vi "Triaxial_Geonor_General.vi"() -> ()   [LabVIEW 2015]
uses:
  <vilib>/Analysis/Matrix/Datatypes/RealMatrix.ctl
  <vilib>/Utility/file.llb/Read From Spreadsheet File (DBL).vi
  <vilib>/Analysis/Matrix/Numeric/Conversions/Array To Matrix - RA.vi
  Variables_Offset.vi
  <vilib>/Analysis/Matrix/NI_Matrix.lvlib
panel:
  in  "BoolSat":bool=TRUE
  in  "BoolBCh":bool=TRUE
  in  "BoolCons":bool=TRUE
  in  "BoolCD":bool=TRUE
  in  "BoolUU":bool=TRUE
  in  "BoolCU":bool=TRUE
  out "Vect Prom Efec":bool
  out "OUTPUT":i32[](array[numeric])
  out "w_4":dbl[][](array[numeric])
  out "w_3s":dbl[][](array[numeric])
  out "Vec_Esfuerzo_principal":dbl[](array[numeric]) format="%.2f"
  out "Vec_Desviador":dbl[](array[numeric]) format="%.2f"
  out "Vec_Promedio_efectivo":dbl[](array[numeric]) format="%.2f"
  out "Vec_Esfuerzo_prom_princ":dbl[](array[numeric]) format="%.2f"
  out "Vec_Esfuerzo_radial":dbl[](array[numeric]) format="%.2f"
  out "Vec_AreaCorr":dbl[](array[numeric]) format="%.2f"
  out "Vec_Deformacionporc":dbl[](array[numeric]) format="%.2f"
  in  "Falla CD":bool
  in  "Falla UU":bool
  in  "Falla CU":bool
  in  "B-Check":bool
  out "Log_tiempo [seg]":ext
  out "Raiz_tiempo [seg]":ext
  out "Tiempo Total[s]":ext
  in  "INICIO":bool
  out "vector B Skepton":dbl[](array[numeric]) format="%.2f"
  out "offset 11":dbl
  out "PresionVol":dbl
  out "LVDT Volumen":bool
  out "LVDT Axial":bool
  out "P. Poros":bool
  out "P. Camara":bool
  out "Celda Carga":bool
  out "vector desp vol":dbl[](array[numeric]) format="%.2f"
  out "TIME RAIZ":dbl[](array[numeric]) format="%.2f"
  out "TIME LOG":dbl[](array[numeric]) format="%.2f"
  out "offset 10":dbl
  out "PresCamara":dbl
  out "offset 9":dbl
  out "PresPoro":dbl
  in  "Consolidación":bool
  in  "Saturación":bool
  out "Boolean":bool
  out "offset 8":dbl
  out "offset 7":dbl
  in  "Offset":bool
  out "Cvol":dbl
  out "Ccarga":dbl
  out "Clvdtax":dbl
  out "Ccamara":dbl
  out "Cporo":dbl
  out "Pvol":dbl
  out "Pcarga":dbl
  out "Plvdtax":dbl
  out "Pcamara":dbl
  out "Pporo":dbl
  out "all rows":dbl[][](array[numeric])
  out "vector poros":dbl[](array[numeric]) format="%.2f"
  out "vector camara":dbl[](array[numeric]) format="%.2f"
  out "vector carga":dbl[](array[numeric]) format="%.2f"
  out "vector desp axial":dbl[](array[numeric]) format="%.2f"
  out "LVDT_AX":dbl
  out "Carga":dbl
  in  "Tab Control":T1(tab)
  in  "Peso [g]":string
  out "Fallando":bool
  out "Consolidando":bool
  out "Saturando":bool
  in  "Muestreo Falla":dbl
  in  "Muestreo Consolidación":dbl
  in  "Muestreo Saturación":dbl
  out "Tiempo Falla [s]":dbl
  out "Tiempo Consolidación [s]":dbl
  out "Tiempo Saturación [s]":dbl
  out "Etapa Actual":string
  in  "Diametro [mm]":string
  in  "Altura [mm]":string
  in  "Filename":path=path "Consolidacion"
  out "path":path
  out "Index":dbl
  out "Cambio de Volumen [mm^3]":dbl(slide) scale=0.0..60.0 scale format="%#_3f"
  out "Presión de Poros [KPa]":dbl(knob) scale=0.0..450.0 scale format="%#_3p"
  out "Desplazamiento Axial [mm]":dbl(slide) scale=0.0..15.0 scale format="%.0p"
  out "Celda de Carga [N]":dbl(knob) scale=0.0..300.0 scale format="%_2p"
  out "Presión de Camara [KPa]":dbl(knob) scale=0.0..450.0 scale format="%#_1f"
  out "B Skempton":dbl
  out "Parametro B camara":dbl
  out "Parametro B Poros":dbl
  in  "Fijar Presiones":bool
  in  "Tab Control 2":enum32{"Grafica A", "Grafica B", "Grafica C"}(tab)
  out "Grafica A":cluster{"X":dbl[], "Y":dbl[]}[](graph)
  in  "OK Button":bool
  out "Grafica B":cluster{"X":dbl[], "Y":dbl[]}[](graph)
  in  "OK Button 2":bool
  out "Grafica C":cluster{"X":dbl[], "Y":dbl[]}[](graph)
  in  "OK Button 3":bool
  in  "Grafica A - Valores en X":string(combo)
  in  "Grafica A - Valores en Y":string(combo)
  in  "Grafica B - Valores en X":string(combo)
  in  "Grafica B - Valores en Y":string(combo)
  in  "Grafica C - Valores en X":string(combo)
  in  "Grafica C - Valores en Y":string(combo)
  out "Error":dbl
  in  "Velocidad mm/min":dbl
  out "V_max":dbl
  out "V_min":dbl
  out "Velocidades":dbl[][](array[numeric])
  out "INPUT":i32[](array[numeric])
  out "OUTPUT":T2
  out "TIME SEC":dbl[](array[numeric]) format="%.2f"
  out "Boolean 2":bool
  out "Tiempo [min]":dbl format="%#_1g"
  in  "stop":bool
  in  "Conect":bool
  # "MOD SAT-CON"
  # "MOD FALLAS"
  # "Sensores Activos"
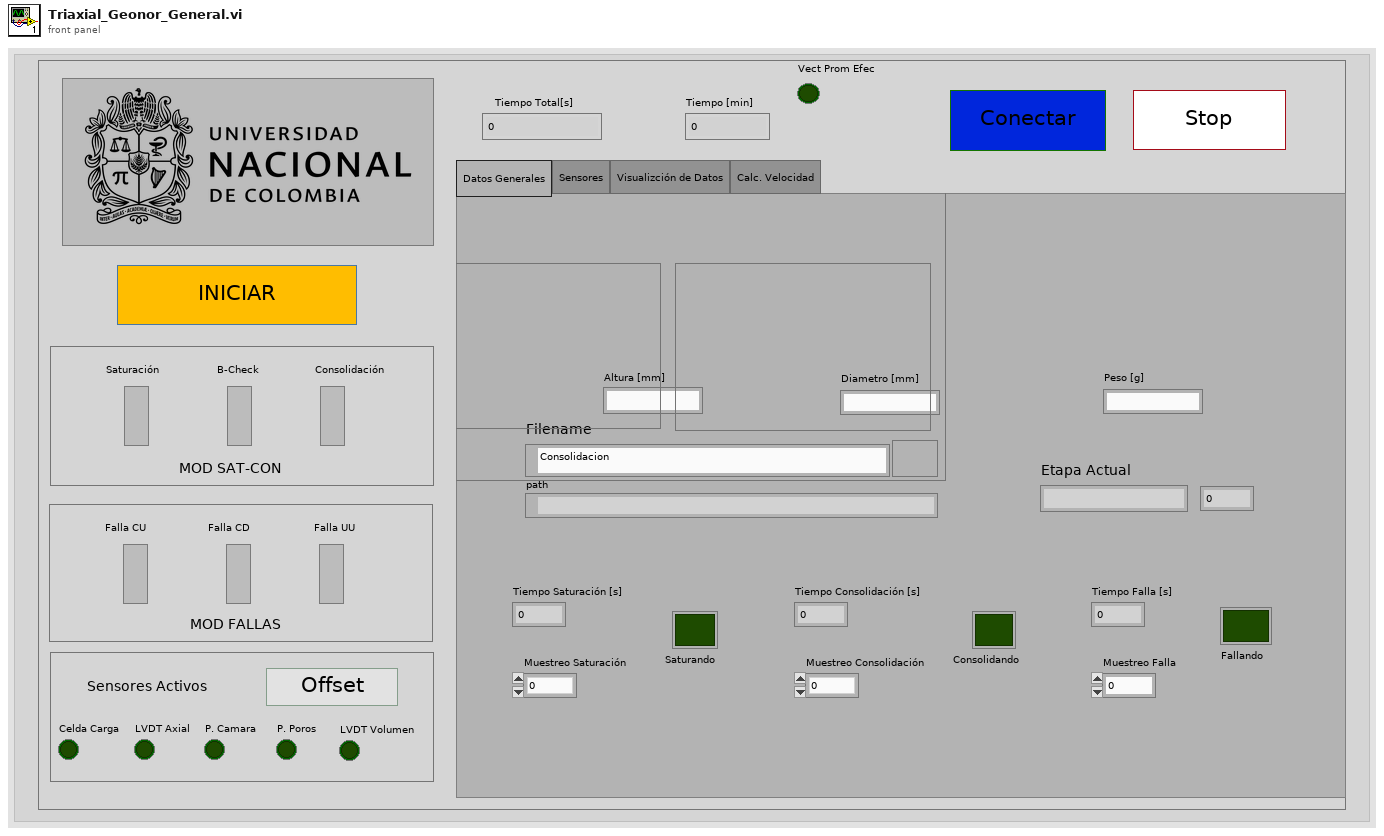
[diagram p1: front panel]
types:
  T1 = enum32{"Datos Generales", "Sensores", "Visualizción de Datos", "Calc. Velocidad"}
  T2 = typedef "NI_Matrix.lvlib/RealMatrix.ctl" = dbl[][]
  T3 = enum16{"open", "open or create", "create or replace", "create", "open (read-only)"}
diagram:
  n1 = flat-sequence {
    frame #0 {
      n2 = while {
        stop <- "Conect" stop-if-true
        n3 = local read "Boolean"() -> (→"Boolean":bool)
      }
      n4 = call "Display Message to User"() -> ()  [unwired: 10 in, 2 out]
      n5 = property on="Tab Control" class="TabCtl (strict)"("PaneHeight"=605) -> (error out=w1:errorcluster)  [unwired: 2 in, 1 out]
      n6 = property on="Tab Control" class="TabCtl (strict)"(error in=w1, "PaneWidth"=890) -> ()  [unwired: 1 in, 2 out]
    }
    frame #1 {
      w8 = FALSE
      w6 = 0.0
      n7 = Initialize Array(0.0, 0 ("dimension size")) -> (→"TIME SEC" →"vector desp axial" →"vector carga" →"vector camara" →"vector poros" →"TIME LOG" →"TIME RAIZ" →"vector desp vol" →"vector B Skepton" →"Vec_Deformacionporc" →"Vec_AreaCorr" →"Vec_Esfuerzo_radial" →"Vec_Esfuerzo_prom_princ" →"Vec_Promedio_efectivo" →"Vec_Desviador" →"Vec_Esfuerzo_principal":dbl[])
      n8 = local write "Saturación"(w8) -> ()
      n9 = local write "Consolidación"(w8) -> ()
      n10 = local write "Falla CU"(w8) -> ()
      n11 = local write "LVDT Axial"(w8) -> ()
      n12 = local write "LVDT Volumen"(w8) -> ()
      n13 = local write "B-Check"(w8) -> ()
      n14 = local write "Celda Carga"(w8) -> ()
      n15 = local write "Consolidando"(w8) -> ()
      n16 = local write "Saturando"(w8) -> ()
      n17 = local write "Falla UU"(w8) -> ()
      n18 = local write "Falla CD"(w8) -> ()
      n19 = local write "Boolean 2"(w8) -> ()
      n20 = local write "P. Camara"(w8) -> ()
      n21 = local write "P. Poros"(w8) -> ()
      n22 = local write "Fallando"(w8) -> ()
      n23 = local write "Parametro B Poros"(w6) -> ()
      n24 = local write "Parametro B camara"(w6) -> ()
      n25 = local write "offset 11"(w6) -> ()
      n26 = local write "offset 7"(w6) -> ()
      n27 = local write "offset 9"(w6) -> ()
      n28 = local write "offset 10"(w6) -> ()
      n29 = local write "B Skempton"(w6) -> ()
      n30 = local write "offset 8"(w6) -> ()
      "Index" <- w6
    }
    frame #2 {
      w16 = ext 0.0 ("x-y*floor(x/y)")
      n31 = Wait (ms)(milliseconds to wait=u32 1000) -> ()  [unwired: 1 out]
      n32 = local write "Tiempo Total[s]"(w16) -> ()
      n33 = local write "Tiempo Consolidación [s]"(w16) -> ()
      n34 = local write "Tiempo Falla [s]"(w16) -> ()
      n35 = local write "Tiempo Saturación [s]"(w16) -> ()
      n36 = Path To String(path="Filename") -> (string=w62:string)
      n37 = Concatenate Strings("C:\\Users\\LAB GEOTECNIA UN IEI\\Desktop\\GEONOR\\GEONOR\\Datos_Ensayo\\", w62) -> (w61:string)
      n38 = String To Path(string=w61) -> (path=w59:path)
      "path" <- w59
      n39 = call-poly <vilib>:"Read From Spreadsheet File.vi"("file path (dialog if empty)"=path "C:/Users/LAB GEOTECNIA UN IEI/Desktop/GEONOR/GEONOR/Archivo_de_calibración.txt") -> ("all rows"=w18:dbl[][])  [unwired: 6 in, 4 out]
      "all rows" <- w18
      n40 = TDMS Open(10:T3."create" ("operation (0:open)"), 11:w59) -> (0:w55:errorcluster, 3:w56:refnum<k34>)  [unwired: 5 in]
      n41 = flat-sequence {
        tunnel: [w69] -> w22
        tunnel: [w68] -> w21
        tunnel: w56 -> [w67]
        tunnel: w55 -> [w66]
        tunnel: w22 -> [w75]
        tunnel: [w74] -> w20
        tunnel: w21 -> [w72]
        tunnel: [w73] -> w19
        tunnel: w20 -> [w81]
        tunnel: [w80] -> w15
        tunnel: w19 -> [w79]
        tunnel: [w78] -> w14
        tunnel: w15 -> [w85]
        tunnel: w14 -> [w87]
        tunnel: [w86] -> w13
        tunnel: [w84] -> w12
        tunnel: w13 -> [w89]
        tunnel: w12 -> [w88]
        frame #0 {
          n42 = TDMS Set Properties(5:"Laboratorio de Geotecnia" ("property name"), 7:"Author" ("property name"), 8:w66, 11:w67) -> (0:w68:errorcluster, 3:w69:refnum<k34>)  [unwired: 2 in, 2 out]
        }
        frame #1 {
          n43 = TDMS Set Properties(5:"Altura [mm]", 7:"Altura [mm]", 8:w72, 11:w75) -> (0:w73:errorcluster, 3:w74:refnum<k34>)  [unwired: 2 in, 2 out]
        }
        frame #2 {
          n44 = TDMS Set Properties(5:"Diametro [mm]", 7:"Diametro [mm]", 8:w79, 11:w81) -> (0:w78:errorcluster, 3:w80:refnum<k34>)  [unwired: 2 in, 2 out]
        }
        frame #3 {
          n45 = TDMS Set Properties(5:"Peso [g]", 7:"Peso [gr]", 8:w87, 11:w85) -> (0:w86:errorcluster, 3:w84:refnum<k34>)  [unwired: 2 in, 2 out]
        }
        frame #4 {
          n46 = TDMS Close(8:w89, 11:w88) -> ()  [unwired: 2 out]
        }
      }
      n47 = Index Array(array=w18, index (row)=1, index (col)=2 ("disabled index (col)")) -> (element=→"Cporo":dbl)
      n48 = Index Array(array=w18, index (row)=1, index (col)=1 ("disabled index (col)")) -> (element=→"Pporo":dbl)
      n49 = Index Array(array=w18, index (row)=2, index (col)=2 ("disabled index (col)")) -> (element=→"Ccamara":dbl)
      n50 = Index Array(array=w18, index (row)=2, index (col)=1 ("disabled index (col)")) -> (element=→"Pcamara":dbl)
      n51 = Index Array(array=w18, index (row)=3, index (col)=2 ("disabled index (col)")) -> (element=→"Clvdtax":dbl)
      n52 = Index Array(array=w18, index (row)=3, index (col)=1 ("disabled index (col)")) -> (element=→"Plvdtax":dbl)
      n53 = Index Array(array=w18, index (row)=4, index (col)=1 ("disabled index (col)")) -> (element=→"Pcarga":dbl)
      n54 = Index Array(array=w18, index (row)=5, index (col)=2 ("disabled index (col)")) -> (element=→"Cvol":dbl)
      n55 = Index Array(array=w18, index (row)=5, index (col)=1 ("disabled index (col)")) -> (element=→"Pvol":dbl)
      n56 = Index Array(array=w18, index (row)=4, index (col)=2 ("disabled index (col)")) -> (element=→"Ccarga":dbl)
      "Boolean 2" <- TRUE
      "Etapa Actual" <- "Esperando Inicio"
      "Error" <- 0.005
    }
    frame #3 {
      n57 = flat-sequence {
        frame #0 {
          n58 = Build Array(24, 33, 34, 40, 46, 47, 50, 60, 63, 71, 72, 82, 96) -> (w92:i32[])
          "INPUT" <- w92
          "OUTPUT" <- w92
          n59 = Array Size(array=w92) -> (size(s)=w93:i32)
          n60 = call-poly <vilib>:"Array To Matrix.vi"("Real 1D Array"=w92) -> ("Real Matrix (Column Vector)"=w91:T2)
          n61 = for {
            N: w93 -> [_]
            tunnel: w93 -> [w113]
            i -> [w111]
            n62 = local read "OUTPUT"() -> (w112:i32[])
            n63 = Index Array(array=w112, index=w111) -> (element=w110:i32)
            n64 = for {
              N: w113 -> [_]
              tunnel: w110 -> [w115]
              tunnel: [w114] -> w107 mode=indexing
              i -> [w119]
              w117 = 0.897  # w_1
              n65 = local read "INPUT"() -> (w120:i32[])
              n66 = Multiply(x=w117, y=w115) -> (x*y=w118:dbl)
              n67 = Index Array(array=w120, index=w119) -> (element=w116:i32)
              n68 = Divide(x=w118, y=w116) -> (x/y=w114:dbl)
            }
            n69 = feedback #1() -> (w108:dbl[][])  [unwired: 1 in]
            n70 = Build Array (concatenate)(w108, w107) -> (w109:dbl[][])
            "w_3s" <- w109
            n71 = feedback-in #1(w109) -> ()
          }
          n72 = Transpose Matrix(1:w91) -> (0:→"OUTPUT":T2)
        }
        frame #1 {
          n73 = local read "w_3s"() -> (w128:dbl[][])
          n74 = Divide(x=w128, y=4) -> (x/y=w126:dbl[][])
          "w_4" <- w126
          n75 = Multiply(x=w126, y=60) -> (x*y=w125:dbl[][])
          n76 = Multiply(x=w125, y=0.02) -> (x*y=w121:dbl[][])
          "Velocidades" <- w121
          n77 = Array Max & Min(array=w121) -> (max value=→"V_max":dbl, min value=→"V_min":dbl)  [unwired: 2 out]
        }
      }
    }
    frame #4 {
      n78 = call "Display Message to User2"() -> ()  [unwired: 10 in, 2 out]
      n79 = while {
        stop <- "INICIO" stop-if-true
      }
    }
    frame #5 {
      n80 = Tick Count (ms)() -> (millisecond timer value=w131:u32)
      n81 = while {
        tunnel: w131 -> [w226]
        stop <- "stop" stop-if-true
        w219 = 1.0
        n82 = Tick Count (ms)() -> (millisecond timer value=w217:u32)
        n83 = global read "Variables_Offset.vi" "Boolean 5"() -> (→"LVDT Volumen":bool)
        n84 = global read "Variables_Offset.vi" "Boolean 4"() -> (→"P. Camara":bool)
        n85 = global read "Variables_Offset.vi" "Boolean 3"() -> (→"P. Poros":bool)
        n86 = global read "Variables_Offset.vi" "Boolean 2"() -> (→"LVDT Axial":bool)
        n87 = global read "Variables_Offset.vi" "Boolean"() -> (→"Celda Carga":bool)
        n88 = case shown="True" "Offset" {
          frame False {
          }
          frame True {
            n89 = vi-ref "Select_Offset.vi"() -> (w882:refnum<vi>)
            n90 = call "Jump.vi"("reference"=w882) -> ()  [unwired: 15 in]
          }
        }
        n91 = Subtract(x=w217, y=w226) -> (x-y=w276:u32)
        n92 = local read "Consolidación"() -> (w210:bool)
        n93 = local read "Consolidación"() -> (w188:bool)
        n94 = local read "Consolidación"() -> (w194:bool)
        n95 = local read "Consolidación"() -> (w213:bool)
        n96 = local read "Consolidación"() -> (w182:bool)
        n97 = call "DAQ Assistant"() -> ("data"=w260:dynamicdata)  [unwired: 16 in, 3 out]
        n98 = local read "Saturación"() -> (w211:bool)
        n99 = local read "Saturación"() -> (w189:bool)
        n100 = local read "Saturación"() -> (w195:bool)
        n101 = local read "Saturación"() -> (w214:bool)
        n102 = local read "Saturación"() -> (w183:bool)
        n103 = local read "B-Check"() -> (w200:bool)
        n104 = local read "B-Check"() -> (w184:bool)
        n105 = local read "B-Check"() -> (w190:bool)
        n106 = local read "B-Check"() -> (w197:bool)
        n107 = local read "B-Check"() -> (w178:bool)
        n108 = local read "Falla CU"() -> (w209:bool)
        n109 = local read "Falla CD"() -> (w202:bool)
        n110 = local read "Falla UU"() -> (w201:bool)
        n111 = local read "Falla CU"() -> (w187:bool)
        n112 = local read "Falla CD"() -> (w186:bool)
        n113 = local read "Falla UU"() -> (w185:bool)
        n114 = local read "Falla CU"() -> (w193:bool)
        n115 = local read "Falla CD"() -> (w192:bool)
        n116 = local read "Falla UU"() -> (w191:bool)
        n117 = local read "Falla CU"() -> (w212:bool)
        n118 = local read "Falla CD"() -> (w199:bool)
        n119 = local read "Falla UU"() -> (w198:bool)
        n120 = local read "Falla CU"() -> (w181:bool)
        n121 = local read "Falla CD"() -> (w180:bool)
        n122 = local read "Falla UU"() -> (w179:bool)
        n123 = Divide(x=w276, y=u32 1000) -> (x/y=w208:dbl)
        "Tiempo Total[s]" <- w208
        n124 = call "Filter3"("Signal"=w260) -> ("Filtered Signal"=w261:dynamicdata)  [unwired: 9 in, 1 out]
        n125 = call "Compuerta_CU.vi"("BCHECK"=w200, "FALLA UU"=w201, "FALLA CD"=w202, "FALLA CU"=w209, "CONSOLIDACION"=w210, "SATURACION"=w211) -> ("Boolean"=w141:bool)  [unwired: 5 in]
        n126 = call "Compuerta_UU.vi"("BCHECK"=w184, "FALLA UU"=w185, "FALLA CD"=w186, "FALLA CU"=w187, "CONSOLIDACION"=w188, "SATURACION"=w189) -> ("Boolean"=w146:bool)  [unwired: 5 in]
        n127 = call "Compuerta_CD.vi"("BCHECK"=w190, "FALLA UU"=w191, "FALLA CD"=w192, "FALLA CU"=w193, "CONSOLIDACION"=w194, "SATURACION"=w195) -> ("Boolean"=w143:bool)  [unwired: 5 in]
        n128 = call "Compuerta_Cons.vi"("BCHECK"=w197, "FALLA UU"=w198, "FALLA CD"=w199, "FALLA CU"=w212, "CONSOLIDACION"=w213, "SATURACION"=w214) -> ("Boolean"=w138:bool)  [unwired: 5 in]
        n129 = call "Compuerta_BCheck.vi"("BCHECK"=w178, "FALLA UU"=w179, "FALLA CD"=w180, "FALLA CU"=w181, "CONSOLIDACION"=w182, "SATURACION"=w183) -> ("Boolean"=w135:bool)  [unwired: 5 in]
        n130 = call "Compuerta_Sat.vi"("BCHECK"="B-Check", "FALLA UU"="Falla UU", "FALLA CD"="Falla CD", "FALLA CU"="Falla CU", "CONSOLIDACION"="Consolidación", "SATURACION"="Saturación") -> ("Boolean"=w151:bool)  [unwired: 5 in]
        n131 = local read "Pcamara"() -> (w248:dbl)
        n132 = local read "Plvdtax"() -> (w257:dbl)
        n133 = local read "Pcarga"() -> (w266:dbl)
        n134 = Compound Arithmetic op=OR(w141, w138, w151, w135, w146, w143) -> (w132:bool)
        "Vect Prom Efec" <- w132
        n135 = Square Root(x=w208) -> (sqrt(x)=→"Raiz_tiempo [seg]":dbl)
        n136 = Not(x=w141) -> (.not. x?=w142:bool)
        n137 = Not(x=w146) -> (.not. x?=w148:bool)
        n138 = Not(x=w143) -> (.not. x?=w145:bool)
        n139 = Not(x=w138) -> (.not. x?=w139:bool)
        n140 = Not(x=w135) -> (.not. x?=w134:bool)
        n141 = Not(x=w151) -> (.not. x?=w150:bool)
        n142 = Split Signals(w261) -> (w262:dynamicdata, w258:dynamicdata, w249:dynamicdata, w245:dynamicdata, w228:dynamicdata)  [unwired: 5 in]
        n143 = local read "Vec_Esfuerzo_prom_princ"() -> (w156:dbl[])
        n144 = Divide(x=w208, y=60.0) -> (x/y=→"Tiempo [min]":dbl)
        n145 = local read "Vec_Promedio_efectivo"() -> (w155:dbl[])
        n146 = Logarithm Base X(1:10.0, 2:w208) -> (0:→"Log_tiempo [seg]":dbl)
        n147 = local read "Vec_Esfuerzo_principal"() -> (w157:dbl[])
        n148 = local read "Vec_Deformacionporc"() -> (w153:dbl[])
        n149 = local read "Vec_Esfuerzo_radial"() -> (w158:dbl[])
        n150 = local read "vector B Skepton"() -> (w152:dbl[])
        n151 = local read "vector desp axial"() -> (w166:dbl[])
        n152 = local read "vector desp vol"() -> (w169:dbl[])
        n153 = local read "Vec_Desviador"() -> (w154:dbl[])
        n154 = local read "vector camara"() -> (w167:dbl[])
        n155 = call "Time CU"("Reset"=w142) -> ("Elapsed Time (s)"=w140:dbl)  [unwired: 11 in, 7 out]
        n156 = call "Time Falla UU"("Reset"=w148) -> ("Elapsed Time (s)"=w147:dbl)  [unwired: 11 in, 7 out]
        n157 = call "Time Falla CD"("Reset"=w145) -> ("Elapsed Time (s)"=w144:dbl)  [unwired: 11 in, 7 out]
        n158 = call "Time Consoli"("Reset"=w139) -> ("Elapsed Time (s)"=w137:dbl)  [unwired: 11 in, 7 out]
        n159 = call "Time B-Chek"("Reset"=w134) -> ("Elapsed Time (s)"=w136:dbl)  [unwired: 11 in, 7 out]
        n160 = call "Time Satur"("Reset"=w150) -> ("Elapsed Time (s)"=w149:dbl)  [unwired: 11 in, 7 out]
        n161 = local read "vector carga"() -> (w165:dbl[])
        n162 = local read "vector poros"() -> (w168:dbl[])
        n163 = local read "TIME RAIZ"() -> (w170:dbl[])
        n164 = local read "TIME LOG"() -> (w171:dbl[])
        n165 = local read "TIME SEC"() -> (w172:dbl[])
        n166 = local read "Ccamara"() -> (w246:dbl)
        n167 = Multiply(x=w258, y=w257) -> (x*y=w259:dynamicdata)
        n168 = Multiply(x=w245, y=w248) -> (x*y=w247:dynamicdata)
        n169 = Multiply(x=w262, y=w266) -> (x*y=w264:dynamicdata)
        n170 = local read "Clvdtax"() -> (w256:dbl)
        n171 = local read "Ccarga"() -> (w265:dbl)
        n172 = local read "Pporo"() -> (w251:dbl)
        n173 = local read "Pvol"() -> (w237:dbl)
        n174 = global read "Variables_Offset.vi" "PresCamaraOff"() -> (w240:bool)
        n175 = global read "Variables_Offset.vi" "LVDTAxOff"() -> (w268:bool)
        n176 = global read "Variables_Offset.vi" "CCargaOff"() -> (w269:bool)
        n177 = case shown="True" w141 {
          tunnel: w140 -> [_ w782]
          frame False {
            n178 = local write "BoolCU"(TRUE) -> ()
          }
          frame True {
            n179 = Initialize Array(0.0, 0 ("dimension size")) -> (w785:dbl[])
            n180 = local write "vector poros"(w785) -> ()
            n181 = local write "Vec_AreaCorr"(w785) -> ()
            n182 = local write "Vec_Deformacionporc"(w785) -> ()
            n183 = local write "Vec_Desviador"(w785) -> ()
            n184 = local write "Vec_Esfuerzo_principal"(w785) -> ()
            n185 = local write "Vec_Esfuerzo_radial"(w785) -> ()
            n186 = local write "Vec_Esfuerzo_prom_princ"(w785) -> ()
            n187 = local write "TIME RAIZ"(w785) -> ()
            n188 = local write "vector carga"(w785) -> ()
            n189 = local write "vector desp axial"(w785) -> ()
            n190 = local write "vector desp vol"(w785) -> ()
            n191 = local write "TIME LOG"(w785) -> ()
            n192 = local write "Vec_Promedio_efectivo"(w785) -> ()
            n193 = local write "TIME SEC"(w785) -> ()
            n194 = local write "vector camara"(w785) -> ()
            n195 = flat-sequence {
              tunnel: w782 -> [w791]
              frame #0 {
                n196 = local read "Index"() -> (w792:dbl)
                n197 = Quotient & Remainder(x=w791, y="Muestreo Falla") -> (x-y*floor(x/y)=w798:dbl)  [unwired: 1 out]
                n198 = Number To Decimal String(number=w792) -> (decimal integer string=w795:string)  [unwired: 1 in]
                n199 = Less?(x=w798, y=0.1) -> (x < y?=w796:bool)
                "Fallando" <- w796
                n200 = Concatenate Strings("Falla CU", w795) -> (w793:string)
                n201 = case shown="True" w796 {
                  tunnel: w793 -> [_ w805]
                  tunnel: w796 -> [_ w804]
                  tunnel: w791 -> [_ w802]
                  frame False {
                  }
                  frame True {
                    n202 = Logarithm Base X(1:10.0, 2:w802) -> (0:w800:dbl)
                    n203 = Square Root(x=w802) -> (sqrt(x)=w801:dbl)
                    n204 = local read "vector carga"() -> (w826:dbl[])
                    n205 = local read "vector desp axial"() -> (w824:dbl[])
                    n206 = local read "vector desp vol"() -> (w818:dbl[])
                    n207 = local read "vector camara"() -> (w821:dbl[])
                    n208 = local read "vector poros"() -> (w819:dbl[])
                    n209 = local read "PresCamara"() -> (w822:dbl)
                    n210 = local read "PresionVol"() -> (w817:dbl)
                    n211 = local read "TIME RAIZ"() -> (w815:dbl[])
                    n212 = local read "TIME LOG"() -> (w816:dbl[])
                    n213 = local read "TIME SEC"() -> (w827:dbl[])
                    n214 = local read "LVDT_AX"() -> (w823:dbl)
                    n215 = local read "PresPoro"() -> (w820:dbl)
                    n216 = local read "Carga"() -> (w825:dbl)
                    n217 = Insert Into Array(array=w815, new element=w801) -> (w811:dbl[])  [unwired: 1 in]
                    n218 = Insert Into Array(array=w827, new element=w802) -> (w813:dbl[])  [unwired: 1 in]
                    n219 = Insert Into Array(array=w818, new element=w817) -> (w806:dbl[])  [unwired: 1 in]
                    n220 = Insert Into Array(array=w824, new element=w823) -> (w809:dbl[])  [unwired: 1 in]
                    n221 = Insert Into Array(array=w826, new element=w825) -> (w810:dbl[])  [unwired: 1 in]
                    n222 = Insert Into Array(array=w816, new element=w800) -> (w812:dbl[])  [unwired: 1 in]
                    n223 = Insert Into Array(array=w821, new element=w822) -> (w807:dbl[])  [unwired: 1 in]
                    n224 = Insert Into Array(array=w819, new element=w820) -> (w808:dbl[])  [unwired: 1 in]
                    n225 = local write "vector desp vol"(w806) -> ()
                    n226 = local write "TIME RAIZ"(w811) -> ()
                    n227 = local write "vector desp axial"(w809) -> ()
                    n228 = local write "vector camara"(w807) -> ()
                    n229 = local write "vector poros"(w808) -> ()
                    n230 = local write "vector carga"(w810) -> ()
                    n231 = local write "TIME SEC"(w813) -> ()
                    n232 = local write "TIME LOG"(w812) -> ()
                    n233 = local read "path"() -> (w814:path)
                    n234 = call "Guardado.vi"("Tiempo"=w813, "Log_Time"=w812, "Raiz_Time"=w811, "Carga"=w810, "LVDT_AX"=w809, "P.Poro"=w808, "P.Camara"=w807, "Path"=w814, "LVDT_Vol"=w806, "Boolean"=w804, "Etapa"=w805) -> ()  [unwired: 8 in, 1 out]
                  }
                }
                n235 = local write "Etapa Actual"(w793) -> ()
                "Tiempo Falla [s]" <- w791
              }
            }
            n236 = flat-sequence {
              frame #0 {
                n237 = local read "Index"() -> (w786:dbl)
                n238 = Increment(x=w786) -> (x+1=w787:dbl)
                n239 = Select(t=w787, s="BoolCU", f=w786) -> (s? t:f=w788:dbl)
                n240 = local write "Index"(w788) -> ()
              }
              frame #1 {
                n241 = local write "BoolCU"(FALSE) -> ()
              }
            }
          }
        }
        n242 = case shown="True" w132 {
          tunnel: w172 -> [_ w352]
          tunnel: w171 -> [_ w350]
          tunnel: "Grafica C - Valores en Y" -> [_ w353]
          tunnel: "Grafica C - Valores en X" -> [_ w354]
          tunnel: "Grafica B - Valores en Y" -> [_ w355]
          tunnel: "Grafica B - Valores en X" -> [_ w356]
          tunnel: "Grafica A - Valores en Y" -> [_ w357]
          tunnel: w170 -> [_ w351]
          tunnel: w169 -> [_ w345]
          tunnel: w168 -> [_ w347]
          tunnel: w167 -> [_ w346]
          tunnel: w166 -> [_ w348]
          tunnel: w165 -> [_ w349]
          tunnel: w152 -> [_ w338]
          tunnel: "Grafica A - Valores en X" -> [_ w364]
          tunnel: w158 -> [_ w344]
          tunnel: w157 -> [_ w343]
          tunnel: w156 -> [_ w342]
          tunnel: w155 -> [_ w341]
          tunnel: w154 -> [_ w340]
          tunnel: w153 -> [_ w339]
          tunnel: w152 -> [_ w337]
          frame False {
          }
          frame True {
            n243 = case shown="\"False\", Default" w356 {
              selector: w356 -> [w476 w481 w482 w484 w486 w488 w490 w493 w495 w497 w499 w501 w503 w505 w507 w509]
              tunnel: [w476 w481 w482 w484 w486 w488 w490 w493 w495 w497 w499 w501 w503 w505 w507 w509] -> w320
              tunnel: [w477 w480 w483 w485 w487 w489 w491 w492 w494 w496 w498 w500 w502 w504 w506 w508] -> w361
              tunnel: w352 -> [_ w480 _ _ _ _ _ _ _ _ _ _ _ _ _ _]
              tunnel: w351 -> [_ _ w483 _ _ _ _ _ _ _ _ _ _ _ _ _]
              tunnel: w350 -> [_ _ _ w485 _ _ _ _ _ _ _ _ _ _ _ _]
              tunnel: w349 -> [_ _ _ _ w487 _ _ _ _ _ _ _ _ _ _ _]
              tunnel: w348 -> [_ _ _ _ _ w489 _ _ _ _ _ _ _ _ _ _]
              tunnel: w347 -> [_ _ _ _ _ _ w491 _ _ _ _ _ _ _ _ _]
              tunnel: w346 -> [_ _ _ _ _ _ _ w492 _ _ _ _ _ _ _ _]
              tunnel: w345 -> [_ _ _ _ _ _ _ _ w494 _ _ _ _ _ _ _]
              tunnel: w344 -> [_ _ _ _ _ _ _ _ _ w496 _ _ _ _ _ _]
              tunnel: w343 -> [_ _ _ _ _ _ _ _ _ _ w498 _ _ _ _ _]
              tunnel: w342 -> [_ _ _ _ _ _ _ _ _ _ _ w500 _ _ _ _]
              tunnel: w341 -> [_ _ _ _ _ _ _ _ _ _ _ _ w502 _ _ _]
              tunnel: w340 -> [_ _ _ _ _ _ _ _ _ _ _ _ _ w504 _ _]
              tunnel: w339 -> [_ _ _ _ _ _ _ _ _ _ _ _ _ _ w506 _]
              tunnel: w337 -> [_ _ _ _ _ _ _ _ _ _ _ _ _ _ _ w508]
              frame "False", Default {
                n244 = Initialize Array(0.0, 0 ("dimension size")) -> (w477:dbl[])
              }
              frame "Tiempo[seg]" {
              }
              frame "Raíz del Tiempo[seg]" {
              }
              frame "Log del Tiempo[seg]" {
              }
              frame "Carga[kN]" {
              }
              frame "LVDT [mm]" {
              }
              frame "Presión de Poros[kPa]" {
              }
              frame "Presión de Camara[kPa]" {
              }
              frame "Cambio de Volumen[mm3]" {
              }
              frame "Esfuerzo Radial[kPa]" {
              }
              frame "Esfuerzo Principal[kPa]" {
              }
              frame "Esfuerzo Promedio[kPa]" {
              }
              frame "Promedio Efectivo[kPa]" {
              }
              frame "Desviador[kPa]" {
              }
              frame "% Deformación" {
              }
              frame "B Skempton" {
              }
            }
            n245 = case shown="\"False\", Default" w355 {
              selector: w355 -> [w442 w447 w448 w450 w452 w454 w456 w459 w461 w463 w465 w467 w469 w471 w473 w475]
              tunnel: [w442 w447 w448 w450 w452 w454 w456 w459 w461 w463 w465 w467 w469 w471 w473 w475] -> w319
              tunnel: [w443 w446 w449 w451 w453 w455 w457 w458 w460 w462 w464 w466 w468 w470 w472 w474] -> w360
              tunnel: w352 -> [_ w446 _ _ _ _ _ _ _ _ _ _ _ _ _ _]
              tunnel: w351 -> [_ _ w449 _ _ _ _ _ _ _ _ _ _ _ _ _]
              tunnel: w350 -> [_ _ _ w451 _ _ _ _ _ _ _ _ _ _ _ _]
              tunnel: w349 -> [_ _ _ _ w453 _ _ _ _ _ _ _ _ _ _ _]
              tunnel: w348 -> [_ _ _ _ _ w455 _ _ _ _ _ _ _ _ _ _]
              tunnel: w347 -> [_ _ _ _ _ _ w457 _ _ _ _ _ _ _ _ _]
              tunnel: w346 -> [_ _ _ _ _ _ _ w458 _ _ _ _ _ _ _ _]
              tunnel: w345 -> [_ _ _ _ _ _ _ _ w460 _ _ _ _ _ _ _]
              tunnel: w344 -> [_ _ _ _ _ _ _ _ _ w462 _ _ _ _ _ _]
              tunnel: w343 -> [_ _ _ _ _ _ _ _ _ _ w464 _ _ _ _ _]
              tunnel: w342 -> [_ _ _ _ _ _ _ _ _ _ _ w466 _ _ _ _]
              tunnel: w341 -> [_ _ _ _ _ _ _ _ _ _ _ _ w468 _ _ _]
              tunnel: w340 -> [_ _ _ _ _ _ _ _ _ _ _ _ _ w470 _ _]
              tunnel: w339 -> [_ _ _ _ _ _ _ _ _ _ _ _ _ _ w472 _]
              tunnel: w337 -> [_ _ _ _ _ _ _ _ _ _ _ _ _ _ _ w474]
              frame "False", Default {
                n246 = Initialize Array(0.0, 0 ("dimension size")) -> (w443:dbl[])
              }
              frame "Tiempo[seg]" {
              }
              frame "Raíz del Tiempo[seg]" {
              }
              frame "Log del Tiempo[seg]" {
              }
              frame "Carga[kN]" {
              }
              frame "LVDT [mm]" {
              }
              frame "Presión de Poros[kPa]" {
              }
              frame "Presión de Camara[kPa]" {
              }
              frame "Cambio de Volumen[mm3]" {
              }
              frame "Esfuerzo Radial[kPa]" {
              }
              frame "Esfuerzo Principal[kPa]" {
              }
              frame "Esfuerzo Promedio[kPa]" {
              }
              frame "Promedio Efectivo[kPa]" {
              }
              frame "Desviador[kPa]" {
              }
              frame "% Deformación" {
              }
              frame "B Skempton" {
              }
            }
            n247 = case shown="\"False\", Default" w364 {
              selector: w364 -> [w544 w549 w550 w552 w554 w556 w558 w561 w563 w565 w567 w569 w571 w573 w575 w577]
              tunnel: [w544 w549 w550 w552 w554 w556 w558 w561 w563 w565 w567 w569 w571 w573 w575 w577] -> w328
              tunnel: [w545 w548 w551 w553 w555 w557 w559 w560 w562 w564 w566 w568 w570 w572 w574 w576] -> w363
              tunnel: w352 -> [_ w548 _ _ _ _ _ _ _ _ _ _ _ _ _ _]
              tunnel: w351 -> [_ _ w551 _ _ _ _ _ _ _ _ _ _ _ _ _]
              tunnel: w350 -> [_ _ _ w553 _ _ _ _ _ _ _ _ _ _ _ _]
              tunnel: w349 -> [_ _ _ _ w555 _ _ _ _ _ _ _ _ _ _ _]
              tunnel: w348 -> [_ _ _ _ _ w557 _ _ _ _ _ _ _ _ _ _]
              tunnel: w347 -> [_ _ _ _ _ _ w559 _ _ _ _ _ _ _ _ _]
              tunnel: w346 -> [_ _ _ _ _ _ _ w560 _ _ _ _ _ _ _ _]
              tunnel: w345 -> [_ _ _ _ _ _ _ _ w562 _ _ _ _ _ _ _]
              tunnel: w344 -> [_ _ _ _ _ _ _ _ _ w564 _ _ _ _ _ _]
              tunnel: w343 -> [_ _ _ _ _ _ _ _ _ _ w566 _ _ _ _ _]
              tunnel: w342 -> [_ _ _ _ _ _ _ _ _ _ _ w568 _ _ _ _]
              tunnel: w341 -> [_ _ _ _ _ _ _ _ _ _ _ _ w570 _ _ _]
              tunnel: w340 -> [_ _ _ _ _ _ _ _ _ _ _ _ _ w572 _ _]
              tunnel: w339 -> [_ _ _ _ _ _ _ _ _ _ _ _ _ _ w574 _]
              tunnel: w338 -> [_ _ _ _ _ _ _ _ _ _ _ _ _ _ _ w576]
              frame "False", Default {
                n248 = Initialize Array(0.0, 0 ("dimension size")) -> (w545:dbl[])
              }
              frame "Tiempo[seg]" {
              }
              frame "Raíz del Tiempo[seg]" {
              }
              frame "Log del Tiempo[seg]" {
              }
              frame "Carga[kN]" {
              }
              frame "LVDT [mm]" {
              }
              frame "Presión de Poros[kPa]" {
              }
              frame "Presión de Camara[kPa]" {
              }
              frame "Cambio de Volumen[mm3]" {
              }
              frame "Esfuerzo Radial[kPa]" {
              }
              frame "Esfuerzo Principal[kPa]" {
              }
              frame "Esfuerzo Promedio[kPa]" {
              }
              frame "Promedio Efectivo[kPa]" {
              }
              frame "Desviador[kPa]" {
              }
              frame "% Deformación" {
              }
              frame "B Skempton" {
              }
            }
            n249 = case shown="\"Presión de Camara[kPa]\"" w357 {
              selector: w357 -> [w510 w515 w516 w518 w520 w522 w524 w527 w529 w531 w533 w535 w537 w539 w541 w543]
              tunnel: [w510 w515 w516 w518 w520 w522 w524 w527 w529 w531 w533 w535 w537 w539 w541 w543] -> w330
              tunnel: [w511 w514 w517 w519 w521 w523 w525 w526 w528 w530 w532 w534 w536 w538 w540 w542] -> w362
              tunnel: w352 -> [_ w514 _ _ _ _ _ _ _ _ _ _ _ _ _ _]
              tunnel: w351 -> [_ _ w517 _ _ _ _ _ _ _ _ _ _ _ _ _]
              tunnel: w350 -> [_ _ _ w519 _ _ _ _ _ _ _ _ _ _ _ _]
              tunnel: w349 -> [_ _ _ _ w521 _ _ _ _ _ _ _ _ _ _ _]
              tunnel: w348 -> [_ _ _ _ _ w523 _ _ _ _ _ _ _ _ _ _]
              tunnel: w347 -> [_ _ _ _ _ _ w525 _ _ _ _ _ _ _ _ _]
              tunnel: w346 -> [_ _ _ _ _ _ _ w526 _ _ _ _ _ _ _ _]
              tunnel: w345 -> [_ _ _ _ _ _ _ _ w528 _ _ _ _ _ _ _]
              tunnel: w344 -> [_ _ _ _ _ _ _ _ _ w530 _ _ _ _ _ _]
              tunnel: w343 -> [_ _ _ _ _ _ _ _ _ _ w532 _ _ _ _ _]
              tunnel: w342 -> [_ _ _ _ _ _ _ _ _ _ _ w534 _ _ _ _]
              tunnel: w341 -> [_ _ _ _ _ _ _ _ _ _ _ _ w536 _ _ _]
              tunnel: w340 -> [_ _ _ _ _ _ _ _ _ _ _ _ _ w538 _ _]
              tunnel: w339 -> [_ _ _ _ _ _ _ _ _ _ _ _ _ _ w540 _]
              tunnel: w338 -> [_ _ _ _ _ _ _ _ _ _ _ _ _ _ _ w542]
              frame "False", Default {
                n250 = Initialize Array(0.0, 0 ("dimension size")) -> (w511:dbl[])
              }
              frame "Tiempo[seg]" {
              }
              frame "Raíz del Tiempo[seg]" {
              }
              frame "Log del Tiempo[seg]" {
              }
              frame "Carga[kN]" {
              }
              frame "LVDT [mm]" {
              }
              frame "Presión de Poros[kPa]" {
              }
              frame "Presión de Camara[kPa]" {
              }
              frame "Cambio de Volumen[mm3]" {
              }
              frame "Esfuerzo Radial[kPa]" {
              }
              frame "Esfuerzo Principal[kPa]" {
              }
              frame "Esfuerzo Promedio[kPa]" {
              }
              frame "Promedio Efectivo[kPa]" {
              }
              frame "Desviador[kPa]" {
              }
              frame "% Deformación" {
              }
              frame "B Skempton" {
              }
            }
            n251 = case shown="\"False\", Default" w354 {
              selector: w354 -> [w408 w413 w414 w416 w418 w420 w422 w425 w427 w429 w431 w433 w435 w437 w439 w441]
              tunnel: [w408 w413 w414 w416 w418 w420 w422 w425 w427 w429 w431 w433 w435 w437 w439 w441] -> w325
              tunnel: [w409 w412 w415 w417 w419 w421 w423 w424 w426 w428 w430 w432 w434 w436 w438 w440] -> w359
              tunnel: w352 -> [_ w412 _ _ _ _ _ _ _ _ _ _ _ _ _ _]
              tunnel: w351 -> [_ _ w415 _ _ _ _ _ _ _ _ _ _ _ _ _]
              tunnel: w350 -> [_ _ _ w417 _ _ _ _ _ _ _ _ _ _ _ _]
              tunnel: w349 -> [_ _ _ _ w419 _ _ _ _ _ _ _ _ _ _ _]
              tunnel: w348 -> [_ _ _ _ _ w421 _ _ _ _ _ _ _ _ _ _]
              tunnel: w347 -> [_ _ _ _ _ _ w423 _ _ _ _ _ _ _ _ _]
              tunnel: w346 -> [_ _ _ _ _ _ _ w424 _ _ _ _ _ _ _ _]
              tunnel: w345 -> [_ _ _ _ _ _ _ _ w426 _ _ _ _ _ _ _]
              tunnel: w344 -> [_ _ _ _ _ _ _ _ _ w428 _ _ _ _ _ _]
              tunnel: w343 -> [_ _ _ _ _ _ _ _ _ _ w430 _ _ _ _ _]
              tunnel: w342 -> [_ _ _ _ _ _ _ _ _ _ _ w432 _ _ _ _]
              tunnel: w341 -> [_ _ _ _ _ _ _ _ _ _ _ _ w434 _ _ _]
              tunnel: w340 -> [_ _ _ _ _ _ _ _ _ _ _ _ _ w436 _ _]
              tunnel: w339 -> [_ _ _ _ _ _ _ _ _ _ _ _ _ _ w438 _]
              tunnel: w337 -> [_ _ _ _ _ _ _ _ _ _ _ _ _ _ _ w440]
              frame "False", Default {
                n252 = Initialize Array(0.0, 0 ("dimension size")) -> (w409:dbl[])
              }
              frame "Tiempo[seg]" {
              }
              frame "Raíz del Tiempo[seg]" {
              }
              frame "Log del Tiempo[seg]" {
              }
              frame "Carga[kN]" {
              }
              frame "LVDT [mm]" {
              }
              frame "Presión de Poros[kPa]" {
              }
              frame "Presión de Camara[kPa]" {
              }
              frame "Cambio de Volumen[mm3]" {
              }
              frame "Esfuerzo Radial[kPa]" {
              }
              frame "Esfuerzo Principal[kPa]" {
              }
              frame "Esfuerzo Promedio[kPa]" {
              }
              frame "Promedio Efectivo[kPa]" {
              }
              frame "Desviador[kPa]" {
              }
              frame "% Deformación" {
              }
              frame "B Skempton" {
              }
            }
            n253 = case shown="\"False\", Default" w353 {
              selector: w353 -> [w374 w379 w380 w382 w384 w386 w388 w391 w393 w395 w397 w399 w401 w403 w405 w407]
              tunnel: [w374 w379 w380 w382 w384 w386 w388 w391 w393 w395 w397 w399 w401 w403 w405 w407] -> w323
              tunnel: [w375 w378 w381 w383 w385 w387 w389 w390 w392 w394 w396 w398 w400 w402 w404 w406] -> w358
              tunnel: w352 -> [_ w378 _ _ _ _ _ _ _ _ _ _ _ _ _ _]
              tunnel: w351 -> [_ _ w381 _ _ _ _ _ _ _ _ _ _ _ _ _]
              tunnel: w350 -> [_ _ _ w383 _ _ _ _ _ _ _ _ _ _ _ _]
              tunnel: w349 -> [_ _ _ _ w385 _ _ _ _ _ _ _ _ _ _ _]
              tunnel: w348 -> [_ _ _ _ _ w387 _ _ _ _ _ _ _ _ _ _]
              tunnel: w347 -> [_ _ _ _ _ _ w389 _ _ _ _ _ _ _ _ _]
              tunnel: w346 -> [_ _ _ _ _ _ _ w390 _ _ _ _ _ _ _ _]
              tunnel: w345 -> [_ _ _ _ _ _ _ _ w392 _ _ _ _ _ _ _]
              tunnel: w344 -> [_ _ _ _ _ _ _ _ _ w394 _ _ _ _ _ _]
              tunnel: w343 -> [_ _ _ _ _ _ _ _ _ _ w396 _ _ _ _ _]
              tunnel: w342 -> [_ _ _ _ _ _ _ _ _ _ _ w398 _ _ _ _]
              tunnel: w341 -> [_ _ _ _ _ _ _ _ _ _ _ _ w400 _ _ _]
              tunnel: w340 -> [_ _ _ _ _ _ _ _ _ _ _ _ _ w402 _ _]
              tunnel: w339 -> [_ _ _ _ _ _ _ _ _ _ _ _ _ _ w404 _]
              tunnel: w337 -> [_ _ _ _ _ _ _ _ _ _ _ _ _ _ _ w406]
              frame "False", Default {
                n254 = Initialize Array(0.0, 0 ("dimension size")) -> (w375:dbl[])
              }
              frame "Tiempo[seg]" {
              }
              frame "Raíz del Tiempo[seg]" {
              }
              frame "Log del Tiempo[seg]" {
              }
              frame "Carga[kN]" {
              }
              frame "LVDT [mm]" {
              }
              frame "Presión de Poros[kPa]" {
              }
              frame "Presión de Camara[kPa]" {
              }
              frame "Cambio de Volumen[mm3]" {
              }
              frame "Esfuerzo Radial[kPa]" {
              }
              frame "Esfuerzo Principal[kPa]" {
              }
              frame "Esfuerzo Promedio[kPa]" {
              }
              frame "Promedio Efectivo[kPa]" {
              }
              frame "Desviador[kPa]" {
              }
              frame "% Deformación" {
              }
              frame "B Skempton" {
              }
            }
            n255 = call "Convert to Dynamic Data4"("Array"=w361) -> ("Dynamic Data Type"=w369:dynamicdata)  [unwired: 3 in]
            n256 = call "Convert to Dynamic Data3"("Array"=w360) -> ("Dynamic Data Type"=w370:dynamicdata)  [unwired: 3 in]
            n257 = call "Convert to Dynamic Data6"("Array"=w363) -> ("Dynamic Data Type"=w365:dynamicdata)  [unwired: 3 in]
            n258 = call "Convert to Dynamic Data5"("Array"=w362) -> ("Dynamic Data Type"=w366:dynamicdata)  [unwired: 3 in]
            n259 = call "Convert to Dynamic Data"("Array"=w359) -> ("Dynamic Data Type"=w372:dynamicdata)  [unwired: 3 in]
            n260 = call "Convert to Dynamic Data2"("Array"=w358) -> ("Dynamic Data Type"=w371:dynamicdata)  [unwired: 3 in]
            n261 = call "Build XY Graph2"("Reset"="OK Button 2", "Y Input"=w370, "X Input"=w369) -> ("error out"=w334:errorcluster, "XY Graph"=→"Grafica B":cluster{"X":dbl[], "Y":dbl[]}[])  [unwired: 7 in]
            n262 = call "Build XY Graph"("Reset"="OK Button 3", "Y Input"=w371, "X Input"=w372) -> ("error out"=w332:errorcluster, "XY Graph"=→"Grafica C":cluster{"X":dbl[], "Y":dbl[]}[])  [unwired: 7 in]
            n263 = call "Build XY Graph3"("Reset"="OK Button", "Y Input"=w366, "X Input"=w365) -> ("error out"=w336:errorcluster, "XY Graph"=→"Grafica A":cluster{"X":dbl[], "Y":dbl[]}[])  [unwired: 7 in]
            n264 = property on="Grafica B" class="XYGraph (strict)"(error in=w334, "XScale.NameLbl.Text"=w320) -> (error out=w333:errorcluster)  [unwired: 1 in, 1 out]
            n265 = property on="Grafica C" class="XYGraph (strict)"(error in=w332, "XScale.NameLbl.Text"=w325) -> (error out=w331:errorcluster)  [unwired: 1 in, 1 out]
            n266 = property on="Grafica A" class="XYGraph (strict)"(error in=w336, "YScale.UnitLabel.Text"=w330) -> (error out=w335:errorcluster)  [unwired: 1 in, 1 out]
            n267 = property on="Grafica B" class="XYGraph (strict)"(error in=w333, "YScale.NameLbl.Text"=w319) -> (error out=w321:errorcluster)  [unwired: 1 in, 1 out]
            n268 = property on="Grafica C" class="XYGraph (strict)"(error in=w331, "YScale.NameLbl.Text"=w323) -> (error out=w324:errorcluster)  [unwired: 1 in, 1 out]
            n269 = property on="Grafica B" class="XYGraph (strict)"(error in=w321, "XScale.UnitLabel.Text"=w320) -> (error out=w322:errorcluster)  [unwired: 1 in, 1 out]
            n270 = property on="Grafica A" class="XYGraph (strict)"(error in=w335, "XScale.UnitLabel.Text"=w328) -> (error out=w327:errorcluster)  [unwired: 1 in, 1 out]
            n271 = property on="Grafica C" class="XYGraph (strict)"(error in=w324, "XScale.UnitLabel.Text"=w325) -> (error out=w326:errorcluster)  [unwired: 1 in, 1 out]
            n272 = property on="Grafica B" class="XYGraph (strict)"(error in=w322, "YScale.UnitLabel.Text"=w319) -> ()  [unwired: 1 in, 2 out]
            n273 = property on="Grafica A" class="XYGraph (strict)"(error in=w327, "YScale.NameLbl.Text"=w330) -> (error out=w329:errorcluster)  [unwired: 1 in, 1 out]
            n274 = property on="Grafica C" class="XYGraph (strict)"(error in=w326, "YScale.UnitLabel.Text"=w323) -> ()  [unwired: 1 in, 2 out]
            n275 = property on="Grafica A" class="XYGraph (strict)"(error in=w329, "XScale.NameLbl.Text"=w328) -> ()  [unwired: 1 in, 2 out]
          }
        }
        n276 = case shown="True" w132 {
          frame False {
          }
          frame True {
            n277 = local read "Diametro [mm]"() -> (w309:string)
            n278 = local read "Altura [mm]"() -> (w312:string)
            n279 = Decimal String To Number(string=w309) -> (number=w310:i32)  [unwired: 2 in, 1 out]
            n280 = Decimal String To Number(string=w312) -> (number=w311:i32)  [unwired: 2 in, 1 out]
            n281 = local read "LVDT_AX"() -> (w313:dbl)
            n282 = Divide(x=w310, y=2) -> (x/y=w306:dbl)
            n283 = local read "Vec_Deformacionporc"() -> (w280:dbl[])
            n284 = Square(x=w306) -> (x^2=w305:dbl)
            n285 = Divide(x=w313, y=w311) -> (x/y=w278:dbl)
            n286 = Insert Into Array(array=w280, new element=w278) -> (w279:dbl[])  [unwired: 1 in]
            n287 = Subtract(x=1, y=w278) -> (x-y=w302:dbl)
            n288 = Multiply(x=w305, y=3.141592653589793) -> (x*y=w304:dbl)
            n289 = local write "Vec_Deformacionporc"(w279) -> ()
            n290 = local read "Vec_AreaCorr"() -> (w315:dbl[])
            n291 = Divide(x=w304, y=w302) -> (x/y=w291:dbl)
            n292 = Insert Into Array(array=w315, new element=w291) -> (w314:dbl[])  [unwired: 1 in]
            n293 = local read "Carga"() -> (w292:dbl)
            n294 = local write "Vec_AreaCorr"(w314) -> ()
            n295 = Divide(x=w292, y=w291) -> (x/y=w293:dbl)
            n296 = local read "PresCamara"() -> (w282:dbl)
            n297 = local read "Vec_Esfuerzo_principal"() -> (w300:dbl[])
            n298 = Add(x=w282, y=w293) -> (x+y=w283:dbl)
            n299 = Multiply(x=w282, y=2) -> (x*y=w290:dbl)
            n300 = local read "Vec_Desviador"() -> (w296:dbl[])
            n301 = local read "Vec_Esfuerzo_prom_princ"() -> (w298:dbl[])
            n302 = Subtract(x=w283, y=w282) -> (x-y=w281:dbl)
            n303 = Add(x=w283, y=w290) -> (x+y=w288:dbl)
            n304 = Insert Into Array(array=w300, new element=w283) -> (w301:dbl[])  [unwired: 1 in]
            n305 = local read "Vec_Promedio_efectivo"() -> (w294:dbl[])
            n306 = local read "PresPoro"() -> (w284:dbl)
            n307 = local write "Vec_Esfuerzo_principal"(w301) -> ()
            n308 = Insert Into Array(array=w296, new element=w281) -> (w297:dbl[])  [unwired: 1 in]
            n309 = Divide(x=w288, y=3) -> (x/y=w285:dbl)
            n310 = local write "Vec_Desviador"(w297) -> ()
            n311 = Subtract(x=w285, y=w284) -> (x-y=w286:dbl)
            n312 = Insert Into Array(array=w298, new element=w285) -> (w299:dbl[])  [unwired: 1 in]
            n313 = local write "Vec_Esfuerzo_prom_princ"(w299) -> ()
            n314 = Insert Into Array(array=w294, new element=w286) -> (w295:dbl[])  [unwired: 1 in]
            n315 = local write "Vec_Promedio_efectivo"(w295) -> ()
          }
        }
        n316 = case shown="True" w146 {
          tunnel: w147 -> [_ w629]
          frame False {
            n317 = local write "BoolUU"(TRUE) -> ()
          }
          frame True {
            n318 = Initialize Array(0.0, 0 ("dimension size")) -> (w628:dbl[])
            n319 = local write "vector poros"(w628) -> ()
            n320 = local write "Vec_AreaCorr"(w628) -> ()
            n321 = local write "Vec_Deformacionporc"(w628) -> ()
            n322 = local write "Vec_Desviador"(w628) -> ()
            n323 = local write "Vec_Esfuerzo_principal"(w628) -> ()
            n324 = local write "Vec_Esfuerzo_prom_princ"(w628) -> ()
            n325 = local write "Vec_Esfuerzo_radial"(w628) -> ()
            n326 = local write "Vec_Promedio_efectivo"(w628) -> ()
            n327 = local write "TIME SEC"(w628) -> ()
            n328 = local write "vector camara"(w628) -> ()
            n329 = local write "vector carga"(w628) -> ()
            n330 = local write "vector desp axial"(w628) -> ()
            n331 = local write "vector desp vol"(w628) -> ()
            n332 = local write "TIME LOG"(w628) -> ()
            n333 = local write "TIME RAIZ"(w628) -> ()
            n334 = flat-sequence {
              frame #0 {
                n335 = local read "Index"() -> (w633:dbl)
                n336 = Increment(x=w633) -> (x+1=w632:dbl)
                n337 = Select(t=w632, s="BoolUU", f=w633) -> (s? t:f=w631:dbl)
                n338 = local write "Index"(w631) -> ()
              }
              frame #1 {
                n339 = local write "BoolUU"(FALSE) -> ()
              }
            }
            n340 = flat-sequence {
              tunnel: w629 -> [w635]
              frame #0 {
                n341 = local write "Tiempo Falla [s]"(w635) -> ()
                n342 = local read "Index"() -> (w636:dbl)
                n343 = local read "Muestreo Falla"() -> (w640:dbl)
                n344 = Number To Decimal String(number=w636) -> (decimal integer string=w639:string)  [unwired: 1 in]
                n345 = Quotient & Remainder(x=w635, y=w640) -> (x-y*floor(x/y)=w642:dbl)  [unwired: 1 out]
                n346 = Concatenate Strings("Falla UU", w639) -> (w637:string)
                n347 = Less?(x=w642, y=0.1) -> (x < y?=w641:bool)
                n348 = local write "Fallando"(w641) -> ()
                n349 = case shown="True" w641 {
                  tunnel: w637 -> [_ w649]
                  tunnel: w641 -> [_ w648]
                  tunnel: w635 -> [_ w646]
                  frame False {
                  }
                  frame True {
                    n350 = Square Root(x=w646) -> (sqrt(x)=w645:dbl)
                    n351 = Logarithm Base X(1:10.0, 2:w646) -> (0:w644:dbl)
                    n352 = local read "vector carga"() -> (w670:dbl[])
                    n353 = local read "vector desp axial"() -> (w668:dbl[])
                    n354 = local read "vector desp vol"() -> (w662:dbl[])
                    n355 = local read "vector camara"() -> (w665:dbl[])
                    n356 = local read "vector poros"() -> (w663:dbl[])
                    n357 = local read "PresCamara"() -> (w666:dbl)
                    n358 = local read "PresionVol"() -> (w661:dbl)
                    n359 = local read "TIME RAIZ"() -> (w659:dbl[])
                    n360 = local read "TIME LOG"() -> (w660:dbl[])
                    n361 = local read "TIME SEC"() -> (w671:dbl[])
                    n362 = local read "LVDT_AX"() -> (w667:dbl)
                    n363 = local read "PresPoro"() -> (w664:dbl)
                    n364 = local read "Carga"() -> (w669:dbl)
                    n365 = Insert Into Array(array=w671, new element=w646) -> (w657:dbl[])  [unwired: 1 in]
                    n366 = Insert Into Array(array=w659, new element=w645) -> (w655:dbl[])  [unwired: 1 in]
                    n367 = Insert Into Array(array=w665, new element=w666) -> (w651:dbl[])  [unwired: 1 in]
                    n368 = Insert Into Array(array=w668, new element=w667) -> (w653:dbl[])  [unwired: 1 in]
                    n369 = Insert Into Array(array=w662, new element=w661) -> (w650:dbl[])  [unwired: 1 in]
                    n370 = Insert Into Array(array=w660, new element=w644) -> (w656:dbl[])  [unwired: 1 in]
                    n371 = Insert Into Array(array=w670, new element=w669) -> (w654:dbl[])  [unwired: 1 in]
                    n372 = Insert Into Array(array=w663, new element=w664) -> (w652:dbl[])  [unwired: 1 in]
                    n373 = local write "vector camara"(w651) -> ()
                    n374 = local write "TIME SEC"(w657) -> ()
                    n375 = local write "TIME RAIZ"(w655) -> ()
                    n376 = local write "vector desp axial"(w653) -> ()
                    n377 = local write "vector desp vol"(w650) -> ()
                    n378 = local read "path"() -> (w658:path)
                    n379 = local write "TIME LOG"(w656) -> ()
                    n380 = local write "vector carga"(w654) -> ()
                    n381 = local write "vector poros"(w652) -> ()
                    n382 = call "Guardado.vi"("Tiempo"=w657, "Log_Time"=w656, "Raiz_Time"=w655, "Carga"=w654, "LVDT_AX"=w653, "P.Poro"=w652, "P.Camara"=w651, "Path"=w658, "LVDT_Vol"=w650, "Boolean"=w648, "Etapa"=w649) -> ()  [unwired: 8 in, 1 out]
                  }
                }
                n383 = local write "Etapa Actual"(w637) -> ()
              }
            }
          }
        }
        n384 = case shown="True" w143 {
          tunnel: w144 -> [_ w582]
          frame False {
            n385 = local write "BoolCD"(TRUE) -> ()
          }
          frame True {
            n386 = Initialize Array(0.0, 0 ("dimension size")) -> (w581:dbl[])
            n387 = local write "vector poros"(w581) -> ()
            n388 = local write "Vec_AreaCorr"(w581) -> ()
            n389 = local write "Vec_Deformacionporc"(w581) -> ()
            n390 = local write "Vec_Desviador"(w581) -> ()
            n391 = local write "Vec_Esfuerzo_principal"(w581) -> ()
            n392 = local write "Vec_Esfuerzo_prom_princ"(w581) -> ()
            n393 = local write "Vec_Esfuerzo_radial"(w581) -> ()
            n394 = local write "Vec_Promedio_efectivo"(w581) -> ()
            n395 = local write "TIME SEC"(w581) -> ()
            n396 = local write "vector camara"(w581) -> ()
            n397 = local write "vector carga"(w581) -> ()
            n398 = local write "vector desp axial"(w581) -> ()
            n399 = local write "vector desp vol"(w581) -> ()
            n400 = local write "TIME LOG"(w581) -> ()
            n401 = local write "TIME RAIZ"(w581) -> ()
            n402 = flat-sequence {
              frame #0 {
                n403 = local read "Index"() -> (w584:dbl)
                n404 = Increment(x=w584) -> (x+1=w585:dbl)
                n405 = Select(t=w585, s="BoolCD", f=w584) -> (s? t:f=w586:dbl)
                n406 = local write "Index"(w586) -> ()
              }
              frame #1 {
                n407 = local write "BoolCD"(FALSE) -> ()
              }
            }
            n408 = flat-sequence {
              tunnel: w582 -> [w588]
              frame #0 {
                n409 = local read "Index"() -> (w589:dbl)
                n410 = local read "Muestreo Falla"() -> (w593:dbl)
                n411 = Number To Decimal String(number=w589) -> (decimal integer string=w592:string)  [unwired: 1 in]
                n412 = local write "Tiempo Falla [s]"(w588) -> ()
                n413 = Quotient & Remainder(x=w588, y=w593) -> (x-y*floor(x/y)=w595:dbl)  [unwired: 1 out]
                n414 = Concatenate Strings("Falla CD", w592) -> (w590:string)
                n415 = Less?(x=w595, y=0.1) -> (x < y?=w594:bool)
                n416 = case shown="True" w594 {
                  tunnel: w590 -> [_ w602]
                  tunnel: w594 -> [_ w601]
                  tunnel: w588 -> [_ w599]
                  frame False {
                  }
                  frame True {
                    n417 = Square Root(x=w599) -> (sqrt(x)=w598:dbl)
                    n418 = Logarithm Base X(1:10.0, 2:w599) -> (0:w597:dbl)
                    n419 = local read "vector carga"() -> (w623:dbl[])
                    n420 = local read "vector desp axial"() -> (w621:dbl[])
                    n421 = local read "vector desp vol"() -> (w615:dbl[])
                    n422 = local read "vector camara"() -> (w618:dbl[])
                    n423 = local read "vector poros"() -> (w616:dbl[])
                    n424 = local read "PresCamara"() -> (w619:dbl)
                    n425 = local read "PresionVol"() -> (w614:dbl)
                    n426 = local read "TIME RAIZ"() -> (w612:dbl[])
                    n427 = local read "TIME LOG"() -> (w613:dbl[])
                    n428 = local read "TIME SEC"() -> (w624:dbl[])
                    n429 = local read "LVDT_AX"() -> (w620:dbl)
                    n430 = local read "PresPoro"() -> (w617:dbl)
                    n431 = local read "Carga"() -> (w622:dbl)
                    n432 = Insert Into Array(array=w612, new element=w598) -> (w608:dbl[])  [unwired: 1 in]
                    n433 = Insert Into Array(array=w624, new element=w599) -> (w610:dbl[])  [unwired: 1 in]
                    n434 = Insert Into Array(array=w613, new element=w597) -> (w609:dbl[])  [unwired: 1 in]
                    n435 = Insert Into Array(array=w621, new element=w620) -> (w606:dbl[])  [unwired: 1 in]
                    n436 = Insert Into Array(array=w615, new element=w614) -> (w603:dbl[])  [unwired: 1 in]
                    n437 = Insert Into Array(array=w618, new element=w619) -> (w604:dbl[])  [unwired: 1 in]
                    n438 = Insert Into Array(array=w616, new element=w617) -> (w605:dbl[])  [unwired: 1 in]
                    n439 = Insert Into Array(array=w623, new element=w622) -> (w607:dbl[])  [unwired: 1 in]
                    n440 = local write "TIME RAIZ"(w608) -> ()
                    n441 = local write "vector desp vol"(w603) -> ()
                    n442 = local write "vector camara"(w604) -> ()
                    n443 = local write "vector desp axial"(w606) -> ()
                    n444 = local write "vector poros"(w605) -> ()
                    n445 = local write "TIME SEC"(w610) -> ()
                    n446 = local write "TIME LOG"(w609) -> ()
                    n447 = local read "path"() -> (w611:path)
                    n448 = local write "vector carga"(w607) -> ()
                    n449 = call "Guardado.vi"("Tiempo"=w610, "Log_Time"=w609, "Raiz_Time"=w608, "Carga"=w607, "LVDT_AX"=w606, "P.Poro"=w605, "P.Camara"=w604, "Path"=w611, "LVDT_Vol"=w603, "Boolean"=w601, "Etapa"=w602) -> ()  [unwired: 8 in, 1 out]
                  }
                }
                n450 = local write "Etapa Actual"(w590) -> ()
                n451 = local write "Fallando"(w594) -> ()
              }
            }
          }
        }
        n452 = case shown="True" w138 {
          tunnel: w137 -> [_ w738]
          frame False {
            n453 = local write "BoolCons"(TRUE) -> ()
          }
          frame True {
            n454 = Initialize Array(0.0, 0 ("dimension size")) -> (w737:dbl[])
            n455 = local write "TIME SEC"(w737) -> ()
            n456 = local write "Vec_AreaCorr"(w737) -> ()
            n457 = local write "Vec_Deformacionporc"(w737) -> ()
            n458 = local write "Vec_Desviador"(w737) -> ()
            n459 = local write "Vec_Esfuerzo_principal"(w737) -> ()
            n460 = local write "Vec_Esfuerzo_prom_princ"(w737) -> ()
            n461 = local write "Vec_Esfuerzo_radial"(w737) -> ()
            n462 = local write "Vec_Promedio_efectivo"(w737) -> ()
            n463 = local write "vector camara"(w737) -> ()
            n464 = local write "vector carga"(w737) -> ()
            n465 = local write "vector desp axial"(w737) -> ()
            n466 = local write "vector desp vol"(w737) -> ()
            n467 = local write "vector poros"(w737) -> ()
            n468 = local write "TIME LOG"(w737) -> ()
            n469 = local write "TIME RAIZ"(w737) -> ()
            n470 = flat-sequence {
              frame #0 {
                n471 = local read "Index"() -> (w742:dbl)
                n472 = Increment(x=w742) -> (x+1=w741:dbl)
                n473 = Select(t=w741, s="BoolCons", f=w742) -> (s? t:f=w740:dbl)
                n474 = local write "Index"(w740) -> ()
              }
              frame #1 {
                n475 = local write "BoolCons"(FALSE) -> ()
              }
            }
            n476 = flat-sequence {
              tunnel: w738 -> [w744]
              frame #0 {
                n477 = local read "Index"() -> (w745:dbl)
                n478 = Quotient & Remainder(x=w744, y="Muestreo Consolidación") -> (x-y*floor(x/y)=w752:dbl)  [unwired: 1 out]
                n479 = Number To Decimal String(number=w745) -> (decimal integer string=w748:string)  [unwired: 1 in]
                n480 = Concatenate Strings("Consolidación", w748) -> (w746:string)
                n481 = Less?(x=w752, y=0.1) -> (x < y?=w749:bool)
                "Consolidando" <- w749
                n482 = local write "Etapa Actual"(w746) -> ()
                n483 = case shown="True" w749 {
                  tunnel: w746 -> [_ w771]
                  tunnel: w749 -> [_ w763]
                  tunnel: w744 -> [_ w761]
                  frame False {
                  }
                  frame True {
                    # "poro\ncamara\nlvdt vol"
                    n484 = Square Root(x=w761) -> (sqrt(x)=w759:dbl)
                    n485 = Logarithm Base X(1:10.0, 2:w761) -> (0:w760:dbl)
                    n486 = local read "vector carga"() -> (w758:dbl[])
                    n487 = local read "TIME SEC"() -> (w780:dbl[])
                    n488 = local read "vector desp axial"() -> (w756:dbl[])
                    n489 = local read "vector desp vol"() -> (w773:dbl[])
                    n490 = local read "vector camara"() -> (w775:dbl[])
                    n491 = local read "vector poros"() -> (w777:dbl[])
                    n492 = local read "PresCamara"() -> (w774:dbl)
                    n493 = local read "PresionVol"() -> (w772:dbl)
                    n494 = local read "TIME RAIZ"() -> (w778:dbl[])
                    n495 = local read "TIME LOG"() -> (w779:dbl[])
                    n496 = local read "PresPoro"() -> (w776:dbl)
                    n497 = local read "LVDT_AX"() -> (w755:dbl)
                    n498 = local read "Carga"() -> (w757:dbl)
                    n499 = Insert Into Array(array=w780, new element=w761) -> (w770:dbl[])  [unwired: 1 in]
                    n500 = local write "TIME SEC"(w770) -> ()
                    n501 = Insert Into Array(array=w778, new element=w759) -> (w768:dbl[])  [unwired: 1 in]
                    n502 = Insert Into Array(array=w777, new element=w776) -> (w767:dbl[])  [unwired: 1 in]
                    n503 = Insert Into Array(array=w773, new element=w772) -> (w765:dbl[])  [unwired: 1 in]
                    n504 = Insert Into Array(array=w756, new element=w755) -> (w753:dbl[])  [unwired: 1 in]
                    n505 = Insert Into Array(array=w775, new element=w774) -> (w766:dbl[])  [unwired: 1 in]
                    n506 = Insert Into Array(array=w758, new element=w757) -> (w754:dbl[])  [unwired: 1 in]
                    n507 = Insert Into Array(array=w779, new element=w760) -> (w769:dbl[])  [unwired: 1 in]
                    n508 = local write "vector poros"(w767) -> ()
                    n509 = local write "vector desp vol"(w765) -> ()
                    n510 = local write "TIME RAIZ"(w768) -> ()
                    n511 = local write "vector camara"(w766) -> ()
                    n512 = local write "vector desp axial"(w753) -> ()
                    n513 = local write "vector carga"(w754) -> ()
                    n514 = local write "TIME LOG"(w769) -> ()
                    n515 = local read "path"() -> (w764:path)
                    n516 = call "Guardado.vi"("Tiempo"=w770, "Log_Time"=w769, "Raiz_Time"=w768, "Carga"=w754, "LVDT_AX"=w753, "P.Poro"=w767, "P.Camara"=w766, "Path"=w764, "LVDT_Vol"=w765, "Boolean"=w763, "Etapa"=w771) -> ()  [unwired: 8 in, 1 out]
                  }
                }
                "Tiempo Consolidación [s]" <- w744
              }
            }
          }
        }
        n517 = case shown="True" w135 {
          tunnel: w136 -> [_ w676]
          frame False {
            n518 = local write "BoolBCh"(TRUE) -> ()
          }
          frame True {
            n519 = Initialize Array(0.0, 0 ("dimension size")) -> (w675:dbl[])
            n520 = local write "TIME RAIZ"(w675) -> ()
            n521 = local write "Vec_Desviador"(w675) -> ()
            n522 = local write "Vec_Esfuerzo_principal"(w675) -> ()
            n523 = local write "vector camara"(w675) -> ()
            n524 = local write "Vec_Esfuerzo_prom_princ"(w675) -> ()
            n525 = local write "vector desp axial"(w675) -> ()
            n526 = local write "Vec_Esfuerzo_radial"(w675) -> ()
            n527 = local write "Vec_Deformacionporc"(w675) -> ()
            n528 = local write "Vec_Promedio_efectivo"(w675) -> ()
            n529 = local write "vector desp vol"(w675) -> ()
            n530 = local write "vector poros"(w675) -> ()
            n531 = local write "TIME SEC"(w675) -> ()
            n532 = local write "vector B Skepton"(w675) -> ()
            n533 = local write "vector carga"(w675) -> ()
            n534 = local write "Vec_AreaCorr"(w675) -> ()
            n535 = local write "TIME LOG"(w675) -> ()
            n536 = flat-sequence {
              frame #0 {
                n537 = local read "Index"() -> (w678:dbl)
                n538 = Increment(x=w678) -> (x+1=w679:dbl)
                n539 = Select(t=w679, s="BoolBCh", f=w678) -> (s? t:f=w680:dbl)
                n540 = local write "Index"(w680) -> ()
              }
              frame #1 {
                n541 = local write "BoolBCh"(FALSE) -> ()
              }
            }
            n542 = flat-sequence {
              tunnel: w676 -> [w682]
              frame #0 {
                n543 = local read "Index"() -> (w683:dbl)
                n544 = local read "Muestreo Saturación"() -> (w688:dbl)
                n545 = Number To Decimal String(number=w683) -> (decimal integer string=w686:string)  [unwired: 1 in]
                n546 = local write "Tiempo Saturación [s]"(w682) -> ()
                n547 = Quotient & Remainder(x=w682, y=w688) -> (x-y*floor(x/y)=w689:dbl)  [unwired: 1 out]
                n548 = Concatenate Strings("B-Check", w686) -> (w684:string)
                n549 = Less?(x=w689, y=0.1) -> (x < y?=w687:bool)
                n550 = local write "Etapa Actual"(w684) -> ()
                n551 = local write "Saturando"(w687) -> ()
                n552 = case shown="True" w687 {
                  tunnel: w684 -> [_ w705]
                  tunnel: w687 -> [_ w704]
                  tunnel: w682 -> [_ w702]
                  frame False {
                  }
                  frame True {
                    n553 = Square Root(x=w702) -> (sqrt(x)=w701:dbl)
                    n554 = Logarithm Base X(1:10.0, 2:w702) -> (0:w700:dbl)
                    n555 = local read "Parametro B camara"() -> (w692:dbl)
                    n556 = local read "Parametro B Poros"() -> (w693:dbl)
                    n557 = local read "PresCamara"() -> (w694:dbl)
                    n558 = local read "PresPoro"() -> (w695:dbl)
                    n559 = local read "vector carga"() -> (w724:dbl[])
                    n560 = Subtract(x=w695, y=w693) -> (x-y=w696:dbl)
                    n561 = Subtract(x=w694, y=w692) -> (x-y=w697:dbl)
                    n562 = local read "vector desp axial"() -> (w722:dbl[])
                    n563 = local read "vector B Skepton"() -> (w699:dbl[])
                    n564 = local read "vector desp vol"() -> (w718:dbl[])
                    n565 = local read "vector camara"() -> (w720:dbl[])
                    n566 = local read "vector poros"() -> (w719:dbl[])
                    n567 = local read "PresionVol"() -> (w717:dbl)
                    n568 = local read "TIME RAIZ"() -> (w715:dbl[])
                    n569 = local read "TIME LOG"() -> (w716:dbl[])
                    n570 = local read "TIME SEC"() -> (w725:dbl[])
                    n571 = local read "LVDT_AX"() -> (w721:dbl)
                    n572 = local read "Carga"() -> (w723:dbl)
                    n573 = Divide(x=w696, y=w697) -> (x/y=w698:dbl)
                    n574 = local write "B Skempton"(w698) -> ()
                    n575 = Insert Into Array(array=w716, new element=w700) -> (w712:dbl[])  [unwired: 1 in]
                    n576 = Insert Into Array(array=w722, new element=w721) -> (w709:dbl[])  [unwired: 1 in]
                    n577 = Insert Into Array(array=w718, new element=w717) -> (w706:dbl[])  [unwired: 1 in]
                    n578 = Insert Into Array(array=w719, new element=w695) -> (w708:dbl[])  [unwired: 1 in]
                    n579 = Insert Into Array(array=w699, new element=w698) -> (w691:dbl[])  [unwired: 1 in]
                    n580 = Insert Into Array(array=w715, new element=w701) -> (w711:dbl[])  [unwired: 1 in]
                    n581 = Insert Into Array(array=w725, new element=w702) -> (w713:dbl[])  [unwired: 1 in]
                    n582 = Insert Into Array(array=w724, new element=w723) -> (w710:dbl[])  [unwired: 1 in]
                    n583 = Insert Into Array(array=w720, new element=w694) -> (w707:dbl[])  [unwired: 1 in]
                    n584 = local write "vector desp vol"(w706) -> ()
                    n585 = local write "vector desp axial"(w709) -> ()
                    n586 = local write "TIME LOG"(w712) -> ()
                    n587 = local write "vector poros"(w708) -> ()
                    n588 = local write "vector B Skepton"(w691) -> ()
                    n589 = local read "path"() -> (w714:path)
                    n590 = local write "TIME RAIZ"(w711) -> ()
                    n591 = local write "vector camara"(w707) -> ()
                    n592 = local write "TIME SEC"(w713) -> ()
                    n593 = local write "vector carga"(w710) -> ()
                    n594 = call "Guardado.vi"("Tiempo"=w713, "Log_Time"=w712, "Raiz_Time"=w711, "Carga"=w710, "LVDT_AX"=w709, "P.Poro"=w708, "P.Camara"=w707, "Path"=w714, "LVDT_Vol"=w706, "Boolean"=w704, "Etapa"=w705, "BSkempton"=w691) -> ()  [unwired: 7 in, 1 out]
                  }
                }
              }
            }
          }
        }
        n595 = case shown="True" w151 {
          tunnel: w149 -> [_ w832]
          frame False {
            n596 = local write "BoolSat"(TRUE) -> ()
          }
          frame True {
            n597 = flat-sequence {
              frame #0 {
                n598 = local read "Index"() -> (w834:dbl)
                n599 = Increment(x=w834) -> (x+1=w835:dbl)
                n600 = Select(t=w835, s="BoolSat", f=w834) -> (s? t:f=w836:dbl)
                n601 = local write "Index"(w836) -> ()
              }
              frame #1 {
                n602 = local write "BoolSat"(FALSE) -> ()
              }
            }
            n603 = Initialize Array(0.0, 0 ("dimension size")) -> (w831:dbl[])
            n604 = local write "vector poros"(w831) -> ()
            n605 = local write "Vec_AreaCorr"(w831) -> ()
            n606 = local write "Vec_Deformacionporc"(w831) -> ()
            n607 = local write "Vec_Desviador"(w831) -> ()
            n608 = local write "Vec_Esfuerzo_principal"(w831) -> ()
            n609 = local write "Vec_Esfuerzo_prom_princ"(w831) -> ()
            n610 = local write "Vec_Esfuerzo_radial"(w831) -> ()
            n611 = local write "Vec_Promedio_efectivo"(w831) -> ()
            n612 = local write "TIME SEC"(w831) -> ()
            n613 = local write "vector B Skepton"(w831) -> ()
            n614 = local write "TIME RAIZ"(w831) -> ()
            n615 = local write "vector camara"(w831) -> ()
            n616 = local write "vector carga"(w831) -> ()
            n617 = local write "vector desp axial"(w831) -> ()
            n618 = local write "vector desp vol"(w831) -> ()
            n619 = local write "TIME LOG"(w831) -> ()
            n620 = flat-sequence {
              tunnel: w832 -> [w838]
              frame #0 {
                n621 = local read "Index"() -> (w839:dbl)
                n622 = Quotient & Remainder(x=w838, y="Muestreo Saturación") -> (x-y*floor(x/y)=w845:dbl)  [unwired: 1 out]
                n623 = Number To Decimal String(number=w839) -> (decimal integer string=w840:string)  [unwired: 1 in]
                n624 = Less?(x=w845, y=0.1) -> (x < y?=w843:bool)
                "Saturando" <- w843
                n625 = Concatenate Strings("Saturación", w840) -> (w841:string)
                n626 = case shown="True" w843 {
                  tunnel: w841 -> [_ w881]
                  tunnel: w843 -> [_ w880]
                  tunnel: w838 -> [_ w879]
                  frame False {
                  }
                  frame True {
                    # "presion poro\npresion camara\nlvdtvolumen"
                    n627 = Square Root(x=w879) -> (sqrt(x)=w858:dbl)
                    n628 = Logarithm Base X(1:10.0, 2:w879) -> (0:w856:dbl)
                    n629 = local read "TIME SEC"() -> (w878:dbl[])
                    n630 = Insert Into Array(array=w878, new element=w879) -> (w872:dbl[])  [unwired: 1 in]
                    n631 = local read "Parametro B camara"() -> (w865:dbl)
                    n632 = local read "Parametro B Poros"() -> (w864:dbl)
                    n633 = local read "PresCamara"() -> (w847:dbl)
                    n634 = local read "PresPoro"() -> (w848:dbl)
                    n635 = local write "TIME SEC"(w872) -> ()
                    n636 = local read "vector carga"() -> (w855:dbl[])
                    n637 = Subtract(x=w848, y=w864) -> (x-y=w862:dbl)
                    n638 = Subtract(x=w847, y=w865) -> (x-y=w863:dbl)
                    n639 = local read "vector desp axial"() -> (w853:dbl[])
                    n640 = local read "vector B Skepton"() -> (w861:dbl[])
                    n641 = local read "vector desp vol"() -> (w874:dbl[])
                    n642 = local read "vector camara"() -> (w875:dbl[])
                    n643 = local read "vector poros"() -> (w876:dbl[])
                    n644 = local read "PresionVol"() -> (w873:dbl)
                    n645 = local read "TIME RAIZ"() -> (w877:dbl[])
                    n646 = local read "TIME LOG"() -> (w857:dbl[])
                    n647 = local read "LVDT_AX"() -> (w852:dbl)
                    n648 = local read "Carga"() -> (w854:dbl)
                    n649 = Divide(x=w862, y=w863) -> (x/y=w849:dbl)
                    "B Skempton" <- w849
                    n650 = Insert Into Array(array=w857, new element=w856) -> (w871:dbl[])  [unwired: 1 in]
                    n651 = Insert Into Array(array=w853, new element=w852) -> (w851:dbl[])  [unwired: 1 in]
                    n652 = Insert Into Array(array=w877, new element=w858) -> (w870:dbl[])  [unwired: 1 in]
                    n653 = Insert Into Array(array=w876, new element=w848) -> (w869:dbl[])  [unwired: 1 in]
                    n654 = Insert Into Array(array=w874, new element=w873) -> (w867:dbl[])  [unwired: 1 in]
                    n655 = Insert Into Array(array=w855, new element=w854) -> (w850:dbl[])  [unwired: 1 in]
                    n656 = Insert Into Array(array=w875, new element=w847) -> (w868:dbl[])  [unwired: 1 in]
                    n657 = Insert Into Array(array=w861, new element=w849) -> (w860:dbl[])  [unwired: 1 in]
                    n658 = local write "TIME LOG"(w871) -> ()
                    n659 = local write "vector desp axial"(w851) -> ()
                    n660 = local read "path"() -> (w866:path)
                    n661 = local write "TIME RAIZ"(w870) -> ()
                    n662 = local write "vector desp vol"(w867) -> ()
                    n663 = local write "vector poros"(w869) -> ()
                    n664 = local write "vector B Skepton"(w860) -> ()
                    n665 = local write "vector carga"(w850) -> ()
                    n666 = local write "vector camara"(w868) -> ()
                    n667 = call "Guardado.vi"("Tiempo"=w872, "Log_Time"=w871, "Raiz_Time"=w870, "Carga"=w850, "LVDT_AX"=w851, "P.Poro"=w869, "P.Camara"=w868, "Path"=w866, "LVDT_Vol"=w867, "Boolean"=w880, "Etapa"=w881, "BSkempton"=w860) -> ()  [unwired: 7 in, 1 out]
                  }
                }
                n668 = local write "Etapa Actual"(w841) -> ()
                "Tiempo Saturación [s]" <- w838
              }
            }
          }
        }
        n669 = Add(x=w259, y=w256) -> (x+y=w244:dynamicdata)
        n670 = Multiply(x=w249, y=w251) -> (x*y=w252:dynamicdata)
        n671 = Add(x=w247, y=w246) -> (x+y=w239:dynamicdata)
        n672 = Multiply(x=w228, y=w237) -> (x*y=w236:dynamicdata)
        n673 = Add(x=w264, y=w265) -> (x+y=w263:dynamicdata)
        n674 = case shown="True" w268 {
          tunnel: [w883 w884] -> w271
          tunnel: w244 -> [w883 w884]
          frame False {
          }
          frame True {
            "offset 8" <- w884
          }
        }
        n675 = local read "Cporo"() -> (w250:dbl)
        n676 = case shown="True" w240 {
          tunnel: [w730 w731] -> w241
          tunnel: w239 -> [w730 w731]
          frame False {
          }
          frame True {
            "offset 10" <- w731
          }
        }
        n677 = case shown="True" w269 {
          tunnel: w263 -> [w885 w886]
          tunnel: [w885 w886] -> w270
          frame False {
          }
          frame True {
            "offset 7" <- w886
          }
        }
        n678 = local read "Cvol"() -> (w235:dbl)
        n679 = global read "Variables_Offset.vi" "PresPoroOff"() -> (w253:bool)
        n680 = global read "Variables_Offset.vi" "LVDTVolOff"() -> (w232:bool)
        n681 = Add(x=w252, y=w250) -> (x+y=w243:dynamicdata)
        n682 = Add(x=w236, y=w235) -> (x+y=w231:dynamicdata)
        n683 = local read "offset 10"() -> (w242:dbl)
        n684 = local read "offset 8"() -> (w272:dbl)
        n685 = local read "offset 7"() -> (w273:dbl)
        n686 = case shown="True" w253 {
          tunnel: [w732 w733] -> w254
          tunnel: w243 -> [w732 w733]
          frame False {
          }
          frame True {
            "offset 9" <- w733
          }
        }
        n687 = case shown="True" w232 {
          tunnel: [w728 w729] -> w233
          tunnel: w231 -> [w728 w729]
          frame False {
          }
          frame True {
            "offset 11" <- w729
          }
        }
        n688 = Subtract(x=w241, y=w242) -> (x-y=w238:dynamicdata)
        n689 = Subtract(x=w271, y=w272) -> (x-y=w224:dynamicdata)
        "LVDT_AX" <- w224
        "Desplazamiento Axial [mm]" <- w224
        n690 = Subtract(x=w270, y=w273) -> (x-y=w225:dynamicdata)
        "Carga" <- w225
        "Celda de Carga [N]" <- w225
        n691 = local read "offset 11"() -> (w234:dbl)
        n692 = local read "offset 9"() -> (w255:dbl)
        n693 = global write "Variables_Offset.vi" "valor 2"(w224) -> ()
        n694 = global write "Variables_Offset.vi" "valor 1"(w225) -> ()
        n695 = Subtract(x=w254, y=w255) -> (x-y=w220:dynamicdata)
        n696 = Subtract(x=w233, y=w234) -> (x-y=w230:dynamicdata)
        n697 = Multiply(x=w220, y=w219) -> (x*y=w218:dynamicdata)
        "PresPoro" <- w218
        "Presión de Poros [KPa]" <- w218
        n698 = Multiply(x=w230, y=1.0) -> (x*y=w133:dynamicdata)
        "PresionVol" <- w133
        "Cambio de Volumen [mm^3]" <- w133
        n699 = Multiply(x=w238, y=w219) -> (x*y=w207:dynamicdata)
        "PresCamara" <- w207
        "Presión de Camara [KPa]" <- w207
        n700 = global write "Variables_Offset.vi" "valor 4"(w207) -> ()
        n701 = global write "Variables_Offset.vi" "valor 3"(w218) -> ()
        n702 = case shown="True" "Fijar Presiones" {
          tunnel: w207 -> [_ w727]
          tunnel: w218 -> [_ w726]
          frame False {
          }
          frame True {
            "Parametro B camara" <- w727
            "Parametro B Poros" <- w726
          }
        }
        n703 = global write "Variables_Offset.vi" "valor 5"(w133) -> ()
      }
    }
  }
